vi "WRAPPER Create Stimulus Session.vi"(8 "Error In":errorcluster, 11 "Stim Player Data In":T1) -> (0 "Error Out":errorcluster, 3 "Stim Player Data Out":T1)   [LabVIEW 2011]
uses:
  Controls/Stim Player Data.ctl
  Controls/Top Level Control.ctl
  <vilib>/NI/AMC/Message Queue.ctl
  <vilib>/NI/AMC/Message.ctl
  <vilib>/NI/Tools/Keyed Array/KeyedArray.ctl
  Controls/ListBox Test Record.ctl
  Controls/DVR of CSV Tests Data.ctl
  Controls/CSVs Tests Data.ctl
  Controls/Test Column Data.ctl
  Controls/Options DVR.ctl
  Controls/Options.ctl
  <vilib>/NI Veristand/Execution/Workspace/WorkspaceAPI.ctl
  NationalInstruments.VeriStand.ClientAPI
  <vilib>/NI Veristand/Execution/SequenceExecutionInterface/Stimulus Profile Session Ref.ctl
  <vilib>/NI Veristand/Execution/ChannelFaultManager/ChannelFaultAPI.ctl
  <vilib>/NI Veristand/Execution/SequenceExecutionInterface/Get All Sequence Names.vi
  <vilib>/NI Veristand/Execution/SequenceExecutionInterface/Open Stimulus Profile Session.vi
  <vilib>/NI Veristand/Execution/SequenceExecutionInterface/Create Sequence Call.vi
  <vilib>/NI Veristand/Execution/SequenceExecutionInterface/Create Sequence Parameter Assignment.vi
  <vilib>/NI Veristand/Execution/SequenceExecutionInterface/Create Sequence Parameter Assignment (Channel).vi
  <vilib>/NI/Tools/Keyed Array/Tools_KeyedArray.lvlib
  <vilib>/NI/AMC/AMC.lvlib
  <vilib>/NI Veristand/Execution/Workspace/NI_VS Workspace ExecutionAPI.lvlib
  <vilib>/NI Veristand/Execution/SequenceExecutionInterface/NI_VS Sequence Execution Interface.lvlib
  <vilib>/NI Veristand/Execution/ChannelFaultManager/NI_VS ChannelFault ExecutionAPI.lvlib
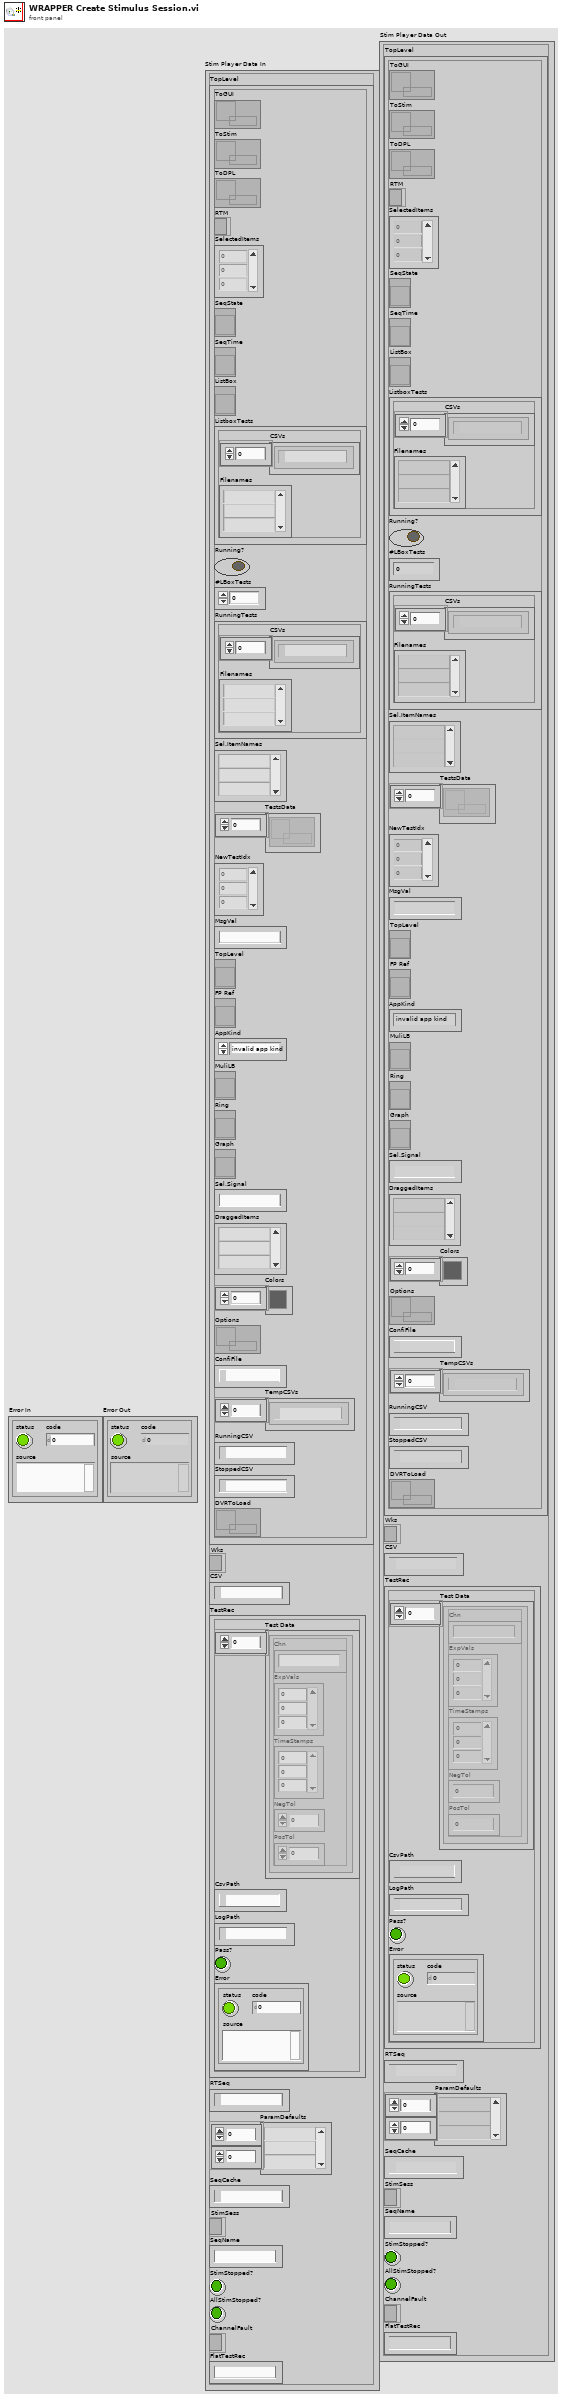
[diagram p1: front panel]
types:
  T1 = typedef "Stim Player Data.ctl" = cluster{"TopLevel":T2, "Wks":T7, "CSV":path, "TestRec":T8, "RTSeq":path, "ParamDefaults":string[][], "SeqCache":path, "StimSess":T10, "SeqName":string, "StimStopped?":bool, "AllStimStopped?":bool, "ChannelFault":T11, "FlatTestRec":string}
  T2 = typedef "Top Level Control.ctl" = cluster{"ToGUI":T3, "ToStim":T3, "ToDPL":T3, "RTM":refnum<k9>, "SelectedItems":i32[], "SeqState":refnum<vi>, "SeqTime":refnum<vi>, "ListBox":refnum<vi>, "ListboxTests":T4, "Running?":bool, "#LBoxTests":i32, "RunningTests":T4, "Sel.ItemNames":string[], "TestsData":T5[], "NewTestIdx":i32[], "MsgVal":string, "TopLevel":refnum<vi>, "FP Ref":refnum<vi>, "AppKind":enum32{"invalid app kind", "Development System", "Run Time System", "Student Edition", "Embedded LabVIEW", "Evaluation", "Custom"}, "MuliLB":refnum<vi>, "Ring":refnum<vi>, "Graph":refnum<vi>, "Sel.Signal":string, "DraggedItems":string[], "Colors":u32[], "Options":T6, "ConfiFile":path, "TempCSVs":path[], "RunningCSV":path, "StoppedCSV":path, "DVRToLoad":T5}
  T3 = typedef "AMC.lvlib/Message Queue.ctl" = refnum<queue>
  T4 = typedef "ListBox Test Record.ctl" = cluster{"CSVs":path[], "Filenames":string[]}
  T5 = typedef "DVR of CSV Tests Data.ctl" = refnum<data-value>
  T6 = typedef "Options DVR.ctl" = refnum<data-value>
  T7 = typedef "NI_VS Workspace ExecutionAPI.lvlib/WorkspaceAPI.ctl" = refnum<k24>
  T8 = typedef "CSVs Tests Data.ctl" = cluster{"Test Data":T9[], "CsvPath":path, "LogPath":path, "Pass?":bool, "Error":errorcluster}
  T9 = typedef "Test Column Data.ctl" = cluster{"Chn":string, "ExpVals":dbl[], "TimeStamps":i64[], "NegTol":dbl, "PosTol":dbl}
  T10 = typedef "NI_VS Sequence Execution Interface.lvlib/Stimulus Profile Session Ref.ctl" = refnum<k24>
  T11 = typedef "NI_VS ChannelFault ExecutionAPI.lvlib/ChannelFaultAPI.ctl" = refnum<k24>
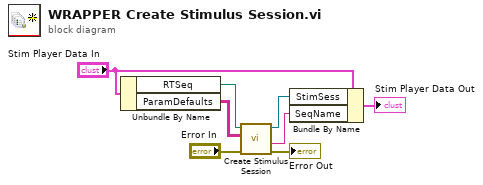
[diagram p0: block diagram]
diagram:
  n1 = Unbundle By Name("Stim Player Data In") -> ("RTSeq"=w6:path, "ParamDefaults"=w5:string[][])
  n2 = call "Create Stimulus Session.vi"("Error In"="Error In", "Parameter Defaults"=w5, "Seq"=w6) -> ("Error Out"=→"Error Out":errorcluster, "Seq Name"=w2:string, "Stim Session Ref"=w3:T10)  [unwired: 6 in]
  n3 = Bundle By Name(cluster="Stim Player Data In", "StimSess"=w3, "SeqName"=w2) -> (→"Stim Player Data Out":T1)
